vi "test Basic Re-reading a future results in error.vi"(8 "error in (no error)":errorcluster, 11 "TestCase in":refnum<class "Futures Tests.lvclass">) -> (0 "error out":errorcluster, 3 "TestCase out":refnum<class "Futures Tests.lvclass">)   [LabVIEW 2017, in "Futures Tests.lvclass"]
uses:
  Futures Tests.lvclass
  <vilib>/Utility/error.llb/Error Cluster From Error Code.vi
  <vilib>/ErrorRing/Error Ring.xnode
  <vilib>/addons/_JKI Toolkits/VI Tester/TestCase.llb/TestCase.lvclass
  Futures/Futures.lvlib
  Futures/Future/Future.lvclass
  Futures/Promise/Promise.lvclass
  C:/Program Files (x86)/National Instruments/LabVIEW 2017/vi.lib/addons/_JKI Toolkits/VI Tester/TestCase.llb/TestCase.lvclass
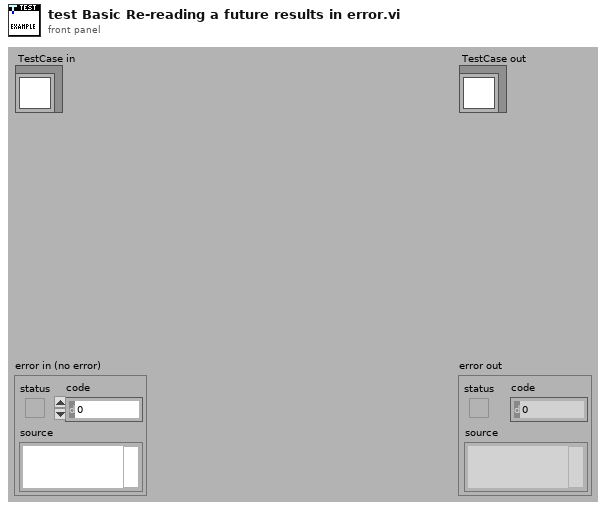
[diagram p1: front panel]
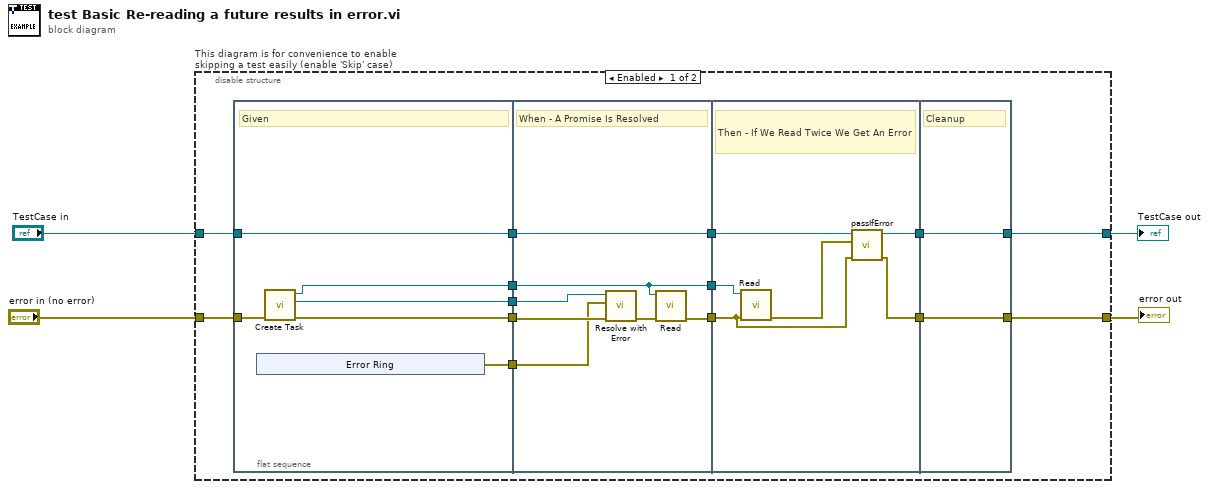
[diagram p0: block diagram]
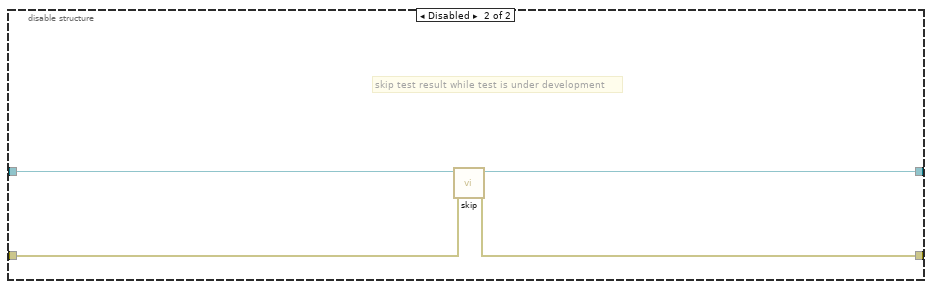
[diagram p2: hidden frame]
diagram:
  n1 = disable-structure "This diagram is for convenience to enable skipping a test easily (enable 'Skip' case)" shown="Enabled" {
    disable-tunnel: "TestCase in" -> [w12 w47]
    disable-tunnel: [w10 w45] -> w1
    disable-tunnel: [w9 w46] -> w3
    disable-tunnel: "error in (no error)" -> [w11 w44]
    frame Enabled {
      n2 = flat-sequence {
        tunnel: w11 -> [w23]
        tunnel: w12 -> [w24]
        tunnel: [w24] -> w18
        tunnel: [w22] -> w17
        tunnel: [w21] -> w8
        tunnel: [w20] -> w6
        tunnel: [w19] -> w5
        tunnel: [w35] -> w16
        tunnel: [w29] -> w15
        tunnel: w18 -> [w35]
        tunnel: w17 -> [w34]
        tunnel: w8 -> [w33]
        tunnel: [w30] -> w7
        tunnel: w6 -> [w30]
        tunnel: w5 -> [w32]
        tunnel: [w40] -> w14
        tunnel: [w39] -> w13
        tunnel: w16 -> [w41]
        tunnel: w15 -> [w36]
        tunnel: w7 -> [w38]
        tunnel: [w42] -> w9
        tunnel: [w43] -> w10
        tunnel: w14 -> [w43]
        tunnel: w13 -> [w42]
        frame #0 {
          # "Given"
          n3 = xnode "Error Ring"() -> ("error out"=w19:errorcluster)
          n4 = call "Create Task.vi"("error in (no error)"=w23) -> ("error out"=w22:errorcluster, "Promise out"=w21:refnum<class "Promise.lvclass">, "Future out"=w20:refnum<class "Future.lvclass">)  [unwired: 8 in]
        }
        frame #1 {
          # "When - A Promise Is Resolved"
          n5 = call "Resolve with Error.vi"("error in (no error)"=w34, "Result"=w32, "Promise in"=w33) -> ("error out"=w31:errorcluster)  [unwired: 8 in]
          n6 = call "Read.vi"("error in (no error)"=w31, "Future in"=w30) -> ("error out"=w29:errorcluster)  [unwired: 6 in, 3 out]
        }
        frame #2 {
          # "Then - If We Read Twice We Get An Error"
          n7 = call "Read.vi"("error in (no error)"=w36, "Future in"=w38) -> ("error out"=w37:errorcluster)  [unwired: 6 in, 3 out]
          n8 = call-dynamic "passIfError.vi"("error in (no error)"=w36, "error"=w37, "TestCase in"=w41) -> ("error out"=w39:errorcluster, "TestCase out"=w40:refnum<class "Futures Tests.lvclass">)  [unwired: 7 in]
        }
        frame #3 {
          # "Cleanup"
        }
      }
    }
    frame Disabled {
      # "skip test result while test is under development"
      n9 = call <vilib>:"skip.vi"("error in (no error)"=w44, "TestCase in"=w47) -> ("error out"=w46:errorcluster, "TestCase out"=w45:refnum<class "Futures Tests.lvclass">)  [unwired: 8 in]
    }
  }
  "error out" <- w3
  "TestCase out" <- w1
